vi "Data process.vi"(8 "error in":errorcluster caption="错误输入", 10 "Data Read":string, 11 "Address":i8=1) -> (0 "error IO":errorcluster, 1 "P":dbl, 2 "I":dbl, 3 "V":dbl)   [LabVIEW 2015]
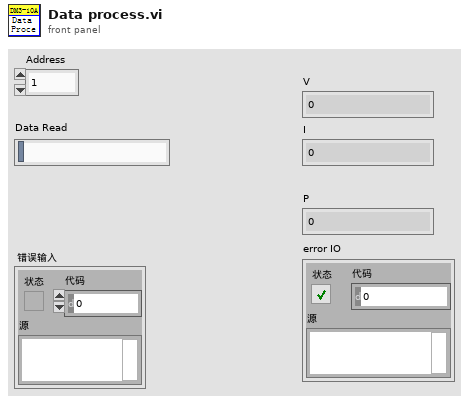
[diagram p1: front panel]
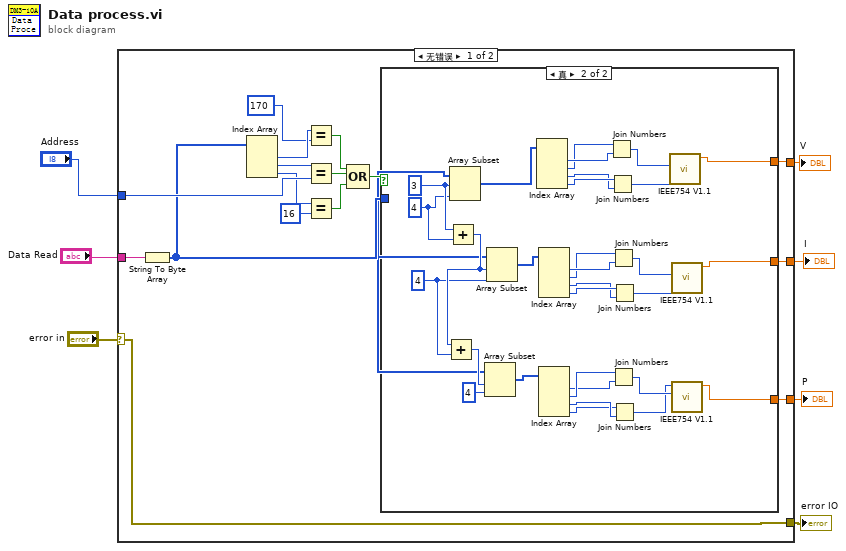
[diagram p0: block diagram]
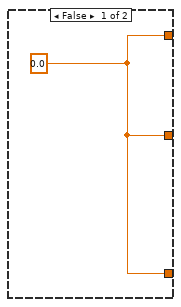
[diagram p2: hidden frame]
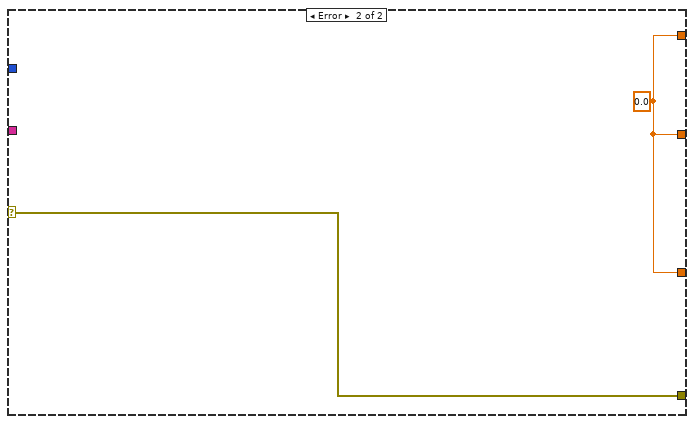
[diagram p3: hidden frame]
diagram:
  n1 = case shown="无错误" "error in" {
    selector: "error in" -> [w22 w57]
    tunnel: "Data Read" -> [w23 _]
    tunnel: [w10 w56] -> w5
    tunnel: [w22 w57] -> w4
    tunnel: "Address" -> [w18 _]
    tunnel: [w9 w56] -> w2
    tunnel: [w8 w56] -> w1
    frame No Error {
      n2 = String To Byte Array(string=w23) -> (unsigned byte array=w11:u8[])
      n3 = Index Array(array=w11) -> (element #1=w21:u8, element #2=w19:u8, element #3=w17:u8)  [unwired: 3 in]
      n4 = Equal?(x=w21, y=u8 170) -> (x = y?=w15:bool)
      n5 = Equal?(x=w19, y=w18) -> (x = y?=w14:bool)
      n6 = Equal?(x=w17, y=u8 16) -> (x = y?=w13:bool)
      n7 = Compound Arithmetic op=OR ("复合运算")(w15, w14, w13) -> (w12:bool)
      n8 = case shown="真" w12 {
        tunnel: w11 -> [_ w33]
        tunnel: [w24 w46] -> w10
        tunnel: [w24 w38] -> w9
        tunnel: [w24 w25] -> w8
        frame False {
          w24 = 0.0 ("输出浮点型")
        }
        frame True {
          w34 = 4 ("长度")
          w55 = 3 ("索引")
          w54 = 4 ("长度")
          n9 = Add(x=w55, y=w54) -> (x+y=w35:i32)
          n10 = Add(x=w35, y=w34) -> (x+y=w37:i32)
          n11 = Array Subset(array=w33, index=w55, length=w54) -> (w53:u8[])
          n12 = Array Subset(array=w33, index=w37, length=4 ("长度")) -> (w26:u8[])
          n13 = Array Subset(array=w33, index=w35, length=w34) -> (w39:u8[])
          n14 = Index Array(array=w53) -> (element #1=w50:u8, element #2=w49:u8, element #3=w51:u8, element #4=w52:u8)  [unwired: 4 in]
          n15 = Index Array(array=w39) -> (element #1=w43:u8, element #2=w42:u8, element #3=w44:u8, element #4=w45:u8)  [unwired: 4 in]
          n16 = Index Array(array=w26) -> (element #1=w29:u8, element #2=w30:u8, element #3=w28:u8, element #4=w27:u8)  [unwired: 4 in]
          n17 = Join Numbers(hi=w49, lo=w50) -> ((hi.lo)=w47:u16)
          n18 = Join Numbers(hi=w52, lo=w51) -> ((hi.lo)=w48:u16)
          n19 = Join Numbers(hi=w42, lo=w43) -> ((hi.lo)=w40:u16)
          n20 = Join Numbers(hi=w30, lo=w29) -> ((hi.lo)=w32:u16)
          n21 = Join Numbers(hi=w45, lo=w44) -> ((hi.lo)=w41:u16)
          n22 = Join Numbers(hi=w27, lo=w28) -> ((hi.lo)=w31:u16)
          n23 = call "IEEE754 V1.1.vi"("低位16"=w47, "高位16"=w48) -> ("输出浮点型"=w46:dbl)  [unwired: 9 in]
          n24 = call "IEEE754 V1.1.vi"("低位16"=w40, "高位16"=w41) -> ("输出浮点型"=w38:dbl)  [unwired: 9 in]
          n25 = call "IEEE754 V1.1.vi"("低位16"=w32, "高位16"=w31) -> ("输出浮点型"=w25:dbl)  [unwired: 9 in]
        }
      }
    }
    frame Error {
      w56 = 0.0 ("输出浮点型")
    }
  }
  "V" <- w5
  "error IO" <- w4
  "I" <- w2
  "P" <- w1
